vi "Destroy.vi"(7 "Sender":refnum<class "Sender.lvclass">) -> (2 "Msg":refnum<class "Msg.lvclass">)   [LabVIEW 2025, in "jettl.lvlib" / "Destroy Msg.lvlib"]
uses:
  Destroy Msg.lvlib
  Destroy Msg/Destroy Msg.lvclass
  C:/git/jettl/src/jettl/jettl/Destroy Msg/Destroy Self Msg/Destroy Msg.lvclass
  C:/git/jettl/src/jettl/jettl/Msg/Msg.lvclass
  Msg/Msg.lvclass
  Sender/Sender/Sender.lvclass
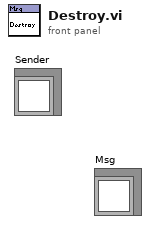
[diagram p1: front panel]
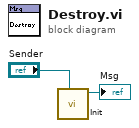
[diagram p0: block diagram]
diagram:
  n1 = call "Init.vi"("Sender"="Sender") -> ("Destroy Msg out"=→"Msg":refnum<class "Destroy Msg.lvclass">)  [unwired: 10 in]
